vi "TDM2TDMSProperties.vi"(0 "tdms file in":refnum<k34>, 5 "Data Object in":refnum<k20>, 7 "group name":string, 9 "channel name":string, 11 "error in (no error)":errorcluster) -> (4 "tdms file out":refnum<k34>, 6 "Data Object out":refnum<k20>, 8 "group name out":string, 10 "channel name out":string, 15 "error out":errorcluster)   [LabVIEW 2020]
doc: "This VI copies named properties from a TDM file, channel group, or channel into corresponding channels in the target TDMS file."
uses:
  <vilib>/Platform/storage/Storage.llb/Get Property (I32).vi
  <vilib>/Platform/storage/Storage.llb/Get Property (DBL).vi
  <vilib>/Platform/storage/Storage.llb/Get Property (Time Stamp).vi
  <vilib>/Platform/storage/Storage.llb/Get Property (String).vi
  <vilib>/Platform/storage/Storage.llb/Get Property (Enum).vi
  <vilib>/Platform/storage/Storage.llb/__loadPropRefList.vi
  <vilib>/Platform/storage/Storage.llb/__loadPropString.vi
  <vilib>/Platform/storage/Storage.llb/__loadPropFloat64.vi
  <vilib>/Platform/storage/Storage.llb/__loadPropInt32.vi
  <vilib>/Platform/storage/Storage.llb/__loadPropTime.vi
  <resource>/objmgr/Storage.rc
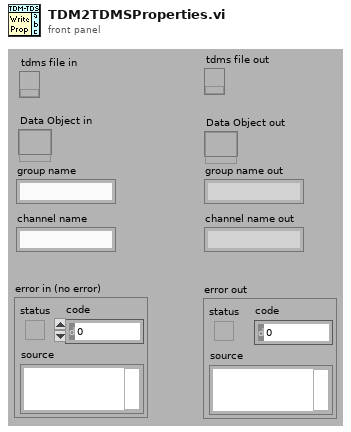
[diagram p1: front panel]
types:
  T1 = typedef "usiPropDef.ctl" = cluster{"name":string, "baseName":string, "refDataType":string, "dimensions":i32, "type":i32, "user defined":bool, "enumStrings":string[], "usiDataType":T2, "specialProp":T3, "Property Source":string, "index":i32}
  T2 = typedef "usiDataType.ctl" = enum16{"eNoTypeUsi", "eInt8Usi", "eInt16Usi", "eInt32Usi", "eInt64Usi", "eUInt8Usi", "eUInt16Usi", "eUInt32Usi", "eUInt64Usi", "eFloat32Usi", "eFloat64Usi", "- 0", "- 1", "- 2", "- 3", "- 4", "- 5", "- 6", "- 7", "- 8", "- 9", "eString8Usi", "eString16Usi", "eStringUsi", "eEnumUsi", "- 10", "- 11", "- 12", "- 13", "- 14", "eTimeUsi", "- 15", "- 16", "- 17", "- 18", "- 19", "- 20", "- 21", "- 22", "- 23", "eInstanceUsi", "eStoreUsi"}
  T3 = typedef "specialProperties.ctl" = enum16{"<Default>", "Channel Values", "AppendReplace", "ChannelFlags", "ValueFlags", "ImplicitExplicit", "InsertIndex", "ValuesCount", "ComparisonOperator", "Cluster", "DAQmx Channel"}
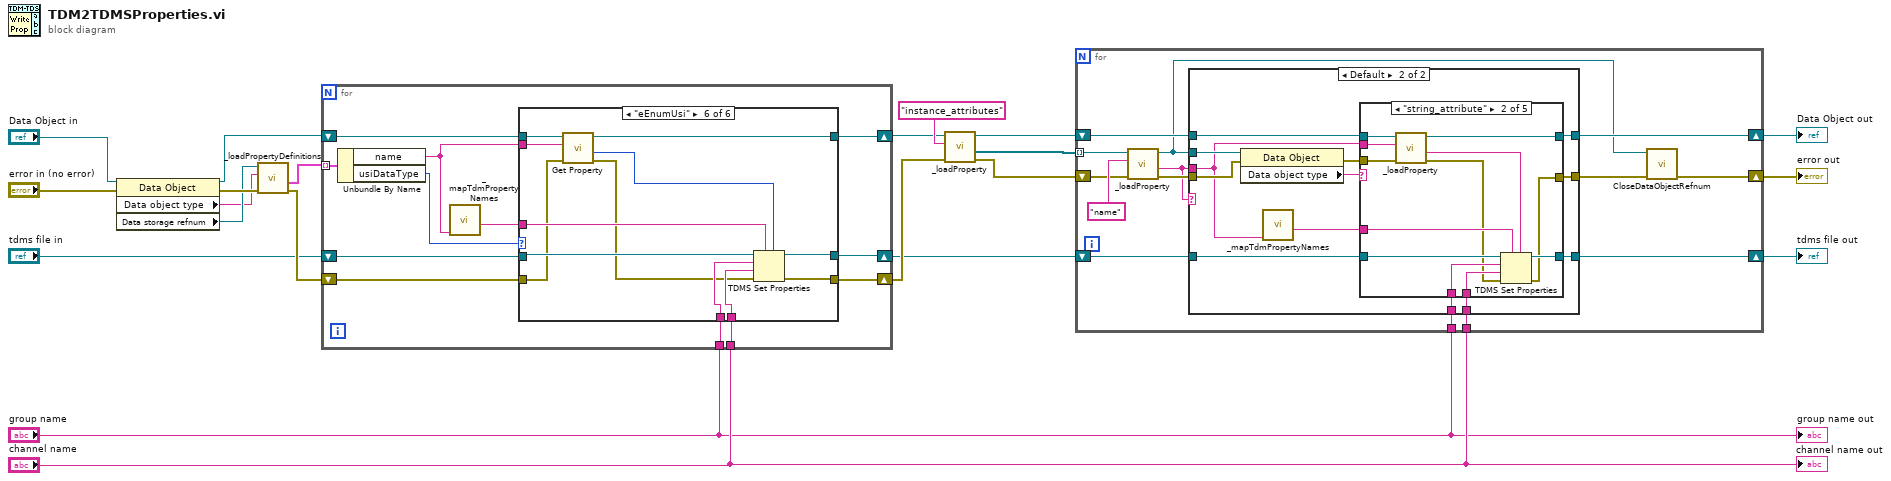
[diagram p0: block diagram]
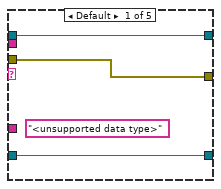
[diagram p3: hidden frame]
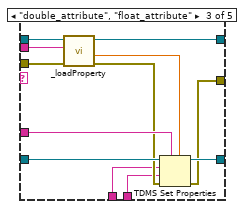
[diagram p4: hidden frame]
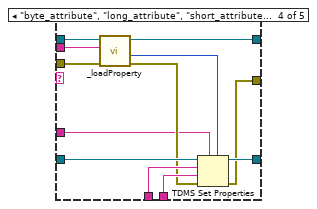
[diagram p5: hidden frame]
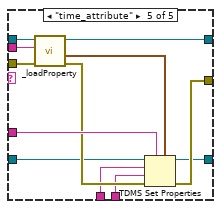
[diagram p6: hidden frame]
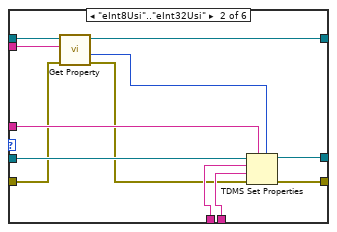
[diagram p8: hidden frame]
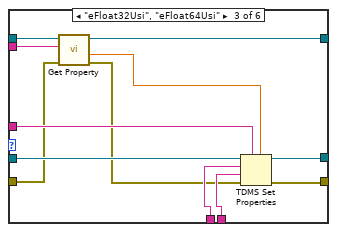
[diagram p9: hidden frame]
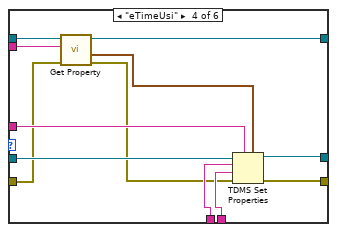
[diagram p10: hidden frame]
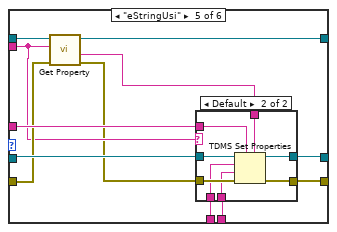
[diagram p11: hidden frame]
diagram:
  n1 = property class="Data Object"(reference="Data Object in", error in="error in (no error)") -> (reference out=w18:refnum<k20>, error out=w21:errorcluster, "Data object type"=w19:string, "Data storage refnum"=w20:refnum<k20>)
  n2 = call <vilib>:"_loadPropertyDefinitions.vi"("error in (no error)"=w21, "Object type"=w19, "storage refnum"=w20) -> ("error out"=w17:errorcluster, "PropertyDefinitions"=w16:T1[])  [unwired: 2 in, 1 out]
  n3 = for {
    shift-right: [w24] -> w8
    shift-left: w17 -> [w31]
    tunnel: w16 -> [w32] mode=indexing
    shift-right: [w26] -> w7
    shift-left: "tdms file in" -> [w29]
    shift-right: [w25] -> w10
    shift-left: w18 -> [w33]
    tunnel: "group name" -> [w23]
    tunnel: "channel name" -> [w22]
    n4 = Unbundle By Name(w32) -> ("name"=w28:string, "usiDataType"=w30:T2)
    n5 = call <vilib>:"_mapTdmPropertyNames.vi"("DNL_Name_in"=w28) -> ("DNL_Mapped_Name_out"=w27:string)  [unwired: 6 in]
    n6 = case shown="\"eEnumUsi\"" w30 {
      tunnel: w28 -> [_ w48 w60 w72 w74 w106]
      tunnel: w31 -> [w34 w41 w53 w62 w78 w99]
      tunnel: w33 -> [w35 w47 w55 w67 w80 w105]
      tunnel: w29 -> [w36 w45 w59 w68 w83 w101]
      tunnel: [w36 w46 w58 w70 w84 w104] -> w26
      tunnel: w27 -> [_ w43 w56 w69 w81 w102]
      tunnel: [w35 w42 w54 w66 w79 w100] -> w25
      tunnel: [w34 w40 w52 w65 w77 w98] -> w24
      tunnel: w23 -> [_ w39 w50 w63 w76 w96]
      tunnel: w22 -> [_ w38 w51 w64 w75 w97]
      frame Default {
      }
      frame "eInt8Usi".."eInt32Usi" {
        n7 = call-poly <vilib>:"Get Property.vi"("error in (no error)"=w41, "Property name"=w48, "storage refnum"=w47) -> ("error out"=w37:errorcluster, "Value"=w44:i32, "storage refnum out"=w42:refnum<k20>)  [unwired: 6 in]
        n8 = TDMS Set Properties(5:w44, 7:w43, 8:w37, 9:w38, 10:w39, 11:w45) -> (0:w40:errorcluster, 3:w46:refnum<k34>)  [unwired: 2 out]
      }
      frame "eFloat32Usi", "eFloat64Usi" {
        n9 = call-poly <vilib>:"Get Property.vi"("error in (no error)"=w53, "Property name"=w60, "storage refnum"=w55) -> ("error out"=w49:errorcluster, "Value"=w57:dbl, "storage refnum out"=w54:refnum<k20>)  [unwired: 6 in]
        n10 = TDMS Set Properties(5:w57, 7:w56, 8:w49, 9:w51, 10:w50, 11:w59) -> (0:w52:errorcluster, 3:w58:refnum<k34>)  [unwired: 2 out]
      }
      frame "eTimeUsi" {
        n11 = call-poly <vilib>:"Get Property.vi"("error in (no error)"=w62, "Property name"=w72, "storage refnum"=w67) -> ("error out"=w61:errorcluster, "Value"=w71:timestamp, "storage refnum out"=w66:refnum<k20>)  [unwired: 6 in]
        n12 = TDMS Set Properties(5:w71, 7:w69, 8:w61, 9:w64, 10:w63, 11:w68) -> (0:w65:errorcluster, 3:w70:refnum<k34>)  [unwired: 2 out]
      }
      frame "eStringUsi" {
        n13 = call-poly <vilib>:"Get Property.vi"("error in (no error)"=w78, "Property name"=w74, "storage refnum"=w80) -> ("error out"=w73:errorcluster, "Value"=w82:string, "storage refnum out"=w79:refnum<k20>)  [unwired: 6 in]
        n14 = case shown="Default" w74 {
          tunnel: [w86 w94] -> w84
          tunnel: w83 -> [w86 w93]
          tunnel: w82 -> [_ w92]
          tunnel: w81 -> [_ w91]
          tunnel: w73 -> [w85 w90]
          tunnel: [w85 w89] -> w77
          tunnel: w76 -> [_ w88]
          tunnel: w75 -> [_ w87]
          frame "name" {
          }
          frame Default {
            n15 = TDMS Set Properties(5:w92, 7:w91, 8:w90, 9:w87, 10:w88, 11:w93) -> (0:w89:errorcluster, 3:w94:refnum<k34>)  [unwired: 2 out]
          }
        }
      }
      frame "eEnumUsi" {
        n16 = call-poly <vilib>:"Get Property.vi"("error in (no error)"=w99, "Property name"=w106, "storage refnum"=w105) -> ("error out"=w95:errorcluster, "Value"=w103:u16, "storage refnum out"=w100:refnum<k20>)  [unwired: 5 in, 1 out]
        n17 = TDMS Set Properties(5:w103, 7:w102, 8:w95, 9:w97, 10:w96, 11:w101) -> (0:w98:errorcluster, 3:w104:refnum<k34>)  [unwired: 2 out]
      }
    }
  }
  n18 = call-poly <vilib>:"_loadProperty.vi"("error in (no error)"=w8, "Property name"="instance_attributes" ("PropertyName"), "storage refnum"=w10) -> ("error out"=w2:errorcluster, "Value"=w14:refnum<k20>[], "dup storage refnum"=w9:refnum<k20>)  [unwired: 6 in]
  n19 = for {
    tunnel: w14 -> [w120] mode=indexing
    shift-right: [w108] -> w4
    shift-left: w2 -> [w118]
    shift-right: [w115] -> w3
    shift-left: w7 -> [w116]
    tunnel: "group name" -> [w114]
    tunnel: "channel name" -> [w113]
    shift-right: [w111] -> w5
    shift-left: w9 -> [w112]
    n20 = call-poly <vilib>:"_loadProperty.vi"("error in (no error)"=w118, "Property name"="name", "storage refnum"=w120) -> ("error out"=w117:errorcluster, "Value"=w110:string, "dup storage refnum"=w107:refnum<k20>)  [unwired: 6 in]
    n21 = case shown="Default" w110 {
      tunnel: [w122 w136] -> w109
      tunnel: w107 -> [_ w135]
      tunnel: w117 -> [w122 w134]
      tunnel: w110 -> [_ w131]
      tunnel: w116 -> [w121 w129]
      tunnel: [w121 w128] -> w115
      tunnel: w114 -> [_ w127]
      tunnel: w113 -> [_ w126]
      tunnel: w112 -> [w123 w125]
      tunnel: [w123 w124] -> w111
      frame "NI_ChannelLength", "NI_DataType" {
      }
      frame Default {
        n22 = property class="Data Object"(reference=w135, error in=w134) -> (error out=w132:errorcluster, "Data object type"=w133:string)  [unwired: 1 out]
        n23 = call <vilib>:"_mapTdmPropertyNames.vi"("DNL_Name_in"=w131) -> ("DNL_Mapped_Name_out"=w130:string)  [unwired: 6 in]
        n24 = case shown="\"string_attribute\"" w133 {
          tunnel: [w139 w141 w155 w165 w181] -> w136
          tunnel: w125 -> [w137 w151 w163 w175 w187]
          tunnel: w131 -> [_ w150 w162 w174 w186]
          tunnel: w132 -> [w139 w149 w161 w173 w185]
          tunnel: w130 -> [_ w145 w157 w167 w184]
          tunnel: w129 -> [w138 w147 w159 w171 w180]
          tunnel: [w138 w148 w160 w172 w179] -> w128
          tunnel: w127 -> [_ w144 w154 w170 w178]
          tunnel: w126 -> [_ w143 w153 w169 w177]
          tunnel: [w137 w140 w152 w164 w176] -> w124
          frame Default {
            (unwired) "<unsupported data type>" ("Value")
          }
          frame "string_attribute" {
            n25 = call-poly <vilib>:"_loadProperty.vi"("error in (no error)"=w149, "Property name"=w150, "storage refnum"=w151) -> ("error out"=w142:errorcluster, "Value"=w146:string, "dup storage refnum"=w140:refnum<k20>)  [unwired: 6 in]
            n26 = TDMS Set Properties(5:w146, 7:w145, 8:w142, 9:w143, 10:w144, 11:w147) -> (0:w141:errorcluster, 3:w148:refnum<k34>)  [unwired: 2 out]
          }
          frame "double_attribute", "float_attribute" {
            n27 = call-poly <vilib>:"_loadProperty.vi"("error in (no error)"=w161, "Property name"=w162, "storage refnum"=w163) -> ("error out"=w156:errorcluster, "Value"=w158:dbl, "dup storage refnum"=w152:refnum<k20>)  [unwired: 6 in]
            n28 = TDMS Set Properties(5:w158, 7:w157, 8:w156, 9:w153, 10:w154, 11:w159) -> (0:w155:errorcluster, 3:w160:refnum<k34>)  [unwired: 2 out]
          }
          frame "byte_attribute", "long_attribute", "short_attribute" {
            n29 = call-poly <vilib>:"_loadProperty.vi"("error in (no error)"=w173, "Property name"=w174, "storage refnum"=w175) -> ("error out"=w168:errorcluster, "Value"=w166:i32, "dup storage refnum"=w164:refnum<k20>)  [unwired: 6 in]
            n30 = TDMS Set Properties(5:w166, 7:w167, 8:w168, 9:w169, 10:w170, 11:w171) -> (0:w165:errorcluster, 3:w172:refnum<k34>)  [unwired: 2 out]
          }
          frame "time_attribute" {
            n31 = call-poly <vilib>:"_loadProperty.vi"("error in (no error)"=w185, "Property name"=w186, "storage refnum"=w187) -> ("error out"=w182:errorcluster, "Value"=w183:timestamp, "dup storage refnum"=w176:refnum<k20>)  [unwired: 6 in]
            n32 = TDMS Set Properties(5:w183, 7:w184, 8:w182, 9:w177, 10:w178, 11:w180) -> (0:w181:errorcluster, 3:w179:refnum<k34>)  [unwired: 2 out]
          }
        }
      }
    }
    n33 = call <vilib>:"CloseDataObjectRefnum.vi"("error in (no error)"=w109, "storage refnum"=w107) -> ("error out"=w108:errorcluster)  [unwired: 9 in]
  }
  "error out" <- w4
  "Data Object out" <- w5
  "tdms file out" <- w3
  "group name out" <- "group name"
  "channel name out" <- "channel name"
